vi "LINX SPI Loopback Benchmark.vi"() -> ()   [LabVIEW 2014, in "LMH-LINX.lvlib"]
doc: "This example demonstrates how to configure the SPI master and do a data loopback test using a LINX device."
uses:
  vi.lib/MakerHub/LINX/LMH-LINX.lvlib
  vi.lib/MakerHub/LINX/Private/Type Defs/Peripherals/SPI/SPI Configuration.ctl
  vi.lib/MakerHub/LINX/Private/Type Defs/Peripherals/SPI/SPI Bit Order.ctl
  vi.lib/MakerHub/LINX/Private/Type Defs/Peripherals/SPI/SPI Mode.ctl
  vi.lib/MakerHub/LINX/Public/Peripherals/SPI/SPI CS Config.ctl
  vi.lib/MakerHub/LINX/Private/Type Defs/Peripherals/SPI/SPI CS Logic Level.ctl
  vi.lib/MakerHub/LINX/Public/Utilities/Open Local.vi
  vi.lib/MakerHub/LINX/Public/Peripherals/SPI/SPI Write Read 1 Frame.vi
panel:
  in  "CS Configuration":T1={"CS Channel"=7, "CS Logic Level"=enum."Active Low"}
  in  "SPI Configuration":T3={"Clock Frequency"=1000000, "Bit Order"=enum."MSb First", "SPI Mode"=enum."Mode 0"}
  in  "SPI Channel":u8
  in  "Benchmark Iterations":i32=1000
  in  "Stop Button":bool
  out "Chart":dbl(graph)=10504.20168067227
  in  "Warmup Iterations":i32=100
  out "Samples Per Second":i32
  out "Read Data":u8[](array[numeric]) format="%.0x"
  in  "Write Data":u8[](array[numeric])=[9, 27, 19, 87] format="%.0x"
  # "SPI Master Settings"
  # "SPI Write / Read \nConfigruation"
  # "SPI Data"
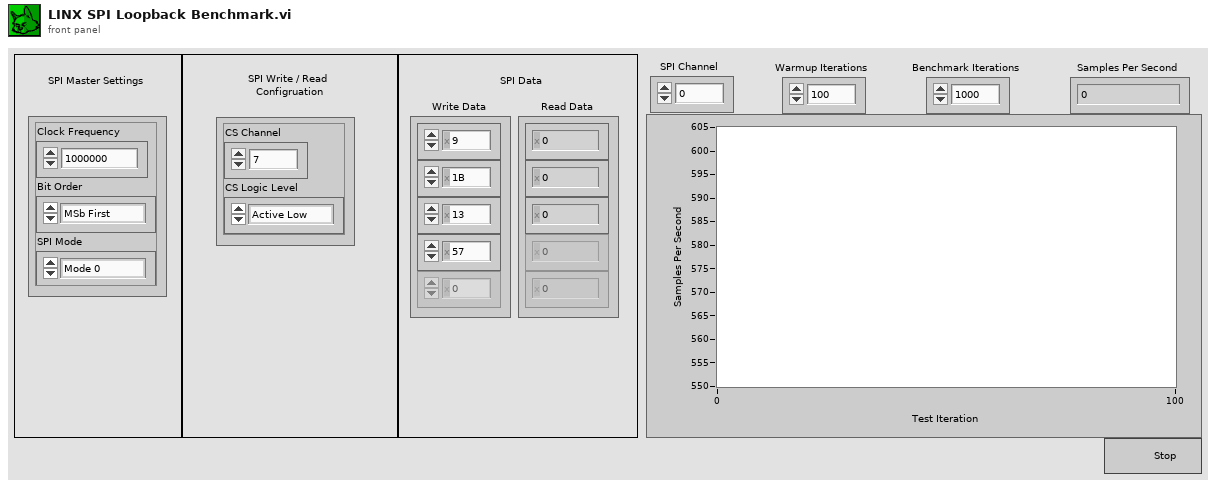
[diagram p1: front panel]
types:
  T1 = typedef "LMH-LINX.lvlib/SPI CS Config.ctl" = cluster{"CS Channel":u8, "CS Logic Level":T2}
  T2 = typedef "LMH-LINX.lvlib/SPI CS Logic Level.ctl" = enum8{"Active Low", "Active High"}
  T3 = typedef "LMH-LINX.lvlib/SPI Configuration.ctl" = cluster{"Clock Frequency":u32, "Bit Order":T4, "SPI Mode":T5}
  T4 = typedef "LMH-LINX.lvlib/SPI Bit Order.ctl" = enum8{"LSb First", "MSb First"}
  T5 = typedef "LMH-LINX.lvlib/SPI Mode.ctl" = enum8{"Mode 0", "Mode 1", "Mode 2", "Mode 3"}
  T6 = typedef "LMH-LINX.lvlib/LINX Ref.ctl" = cluster{"IO":T7, "Interface":T8, "LINX Device Config":T9}
  T7 = typedef "LMH-LINX.lvlib/Platform.ctl" = enum16{"Remote", "Local"}
  T8 = typedef "LMH-LINX.lvlib/Interface.ctl" = enum16{"Serial", "TCP"}
  T9 = typedef "LMH-LINX.lvlib/Device.lvlib/LINX Device Config.ctl" = cluster{"Interface":T8, "COM Port":refnum<visa-resource-name>, "TCP Configuration":T10, "Device Family":u8, "Device ID":u8, "Device Name":string, "TCP Ref":refnum<k5>, "Channels":T11}
  T10 = typedef "LMH-LINX.lvlib/Device.lvlib/TCP Config.ctl" = cluster{"IP Address":string, "Port":u16}
  T11 = typedef "LMH-LINX.lvlib/Channels.ctl" = cluster{"DI":u8[], "DO":u8[], "AI":u8[], "AO":u8[], "PWM":u8[], "QE":u8[], "UART":u8[], "I2C 2":u8[], "SPI":u8[], "CAN":u8[], "Servo":u8[], "AI Ref (V)":dbl, "AI Resolution (Bits)":u8, "AO Ref (V)":dbl, "AO Resolution (Bits)":u8}
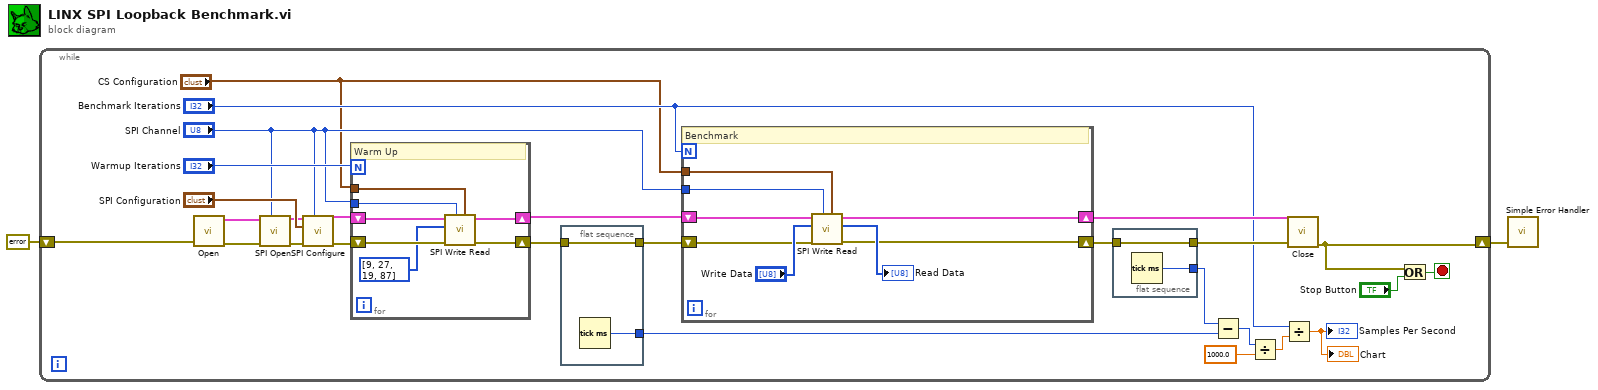
[diagram p0: block diagram]
diagram:
  n1 = while {
    shift-right: [w22] -> w2
    shift-left: errorcluster {"status"=FALSE, "code"=0, "source"=""} ("Error Out") -> [w7]
    stop <- w15 stop-if-true
    n2 = call-poly "Open.vi"("Error In"=w7) -> ("Error Out"=w13:errorcluster, "LINX Resource"=w10:T6)  [unwired: 8 in, 1 out]
    n3 = call "SPI Open.vi"("SPI Channel (0)"="SPI Channel", "Error In"=w13, "LINX Resource"=w10) -> ("Error Out"=w12:errorcluster, "LINX Resource"=w11:T6)  [unwired: 7 in]
    n4 = call "SPI Configure.vi"("SPI Channel (0)"="SPI Channel", "Error In"=w12, "SPI Configuration"="SPI Configuration", "LINX Resource"=w11) -> ("Error Out"=w9:errorcluster, "LINX Resource"=w8:T6)  [unwired: 5 in, 1 out]
    n5 = for {
      N: "Warmup Iterations" -> [_]
      shift-right: [w31] -> w24
      shift-left: w8 -> [w36]
      shift-right: [w32] -> w25
      shift-left: w9 -> [w35]
      tunnel: "SPI Channel" -> [w34]
      tunnel: "CS Configuration" -> [w30]
      # "Warm Up"
      n6 = call-poly "SPI Write Read.vi"("CS Configuration"=w30, "SPI Channel (0)"=w34, "Error In"=w35, "Data"=u8[] [9, 27, 19, 87] ("Write Data"), "LINX Resource"=w36) -> ("Error Out"=w32:errorcluster, "LINX Resource"=w31:T6)  [unwired: 4 in, 1 out]
    }
    n7 = flat-sequence {
      tunnel: [w48] -> w28
      tunnel: w25 -> [w48]
      tunnel: [w47] -> w4
      frame #0 {
        n8 = Tick Count (ms)() -> (millisecond timer value=w47:u32)
      }
    }
    n9 = for {
      N: "Benchmark Iterations" -> [_]
      shift-right: [w39] -> w29
      shift-left: w24 -> [w42]
      shift-right: [w40] -> w27
      shift-left: w28 -> [w41]
      tunnel: "SPI Channel" -> [w37]
      tunnel: "CS Configuration" -> [w38]
      # "Benchmark"
      n10 = call-poly "SPI Write Read.vi"("CS Configuration"=w38, "SPI Channel (0)"=w37, "Error In"=w41, "Data"="Write Data", "LINX Resource"=w42) -> ("Error Out"=w40:errorcluster, "Read Data"=→"Read Data":u8[], "LINX Resource"=w39:T6)  [unwired: 4 in]
    }
    n11 = flat-sequence {
      tunnel: [w46] -> w26
      tunnel: w27 -> [w46]
      tunnel: [w45] -> w18
      frame #0 {
        n12 = Tick Count (ms)() -> (millisecond timer value=w45:u32)
      }
    }
    n13 = Subtract(x=w18, y=w4) -> (x-y=w20:u32)
    n14 = Divide(x=w20, y=1000.0) -> (x/y=w3:dbl)
    n15 = Divide(x="Benchmark Iterations", y=w3) -> (x/y=→"Chart" →"Samples Per Second":dbl)
    n16 = call "Close.vi"("Error In"=w26, "LINX Resource"=w29) -> ("Error Out"=w22:errorcluster)  [unwired: 9 in]
    n17 = Or(x=w22, y="Stop Button") -> (x .or. y?=w15:bool)
  }
  n18 = call <vilib>:"Simple Error Handler.vi"("error in (no error)"=w2) -> ()  [unwired: 4 in, 5 out]
